vi "_Handle Error.vi"(4 "error in (no error)":errorcluster, 6 "Display Warning (T)":bool=TRUE, 7 "Display Error (T)":bool=TRUE) -> (3 "error?":bool)   [LabVIEW 2015]
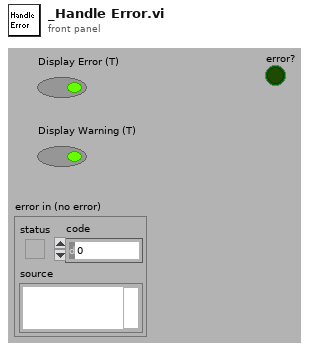
[diagram p1: front panel]
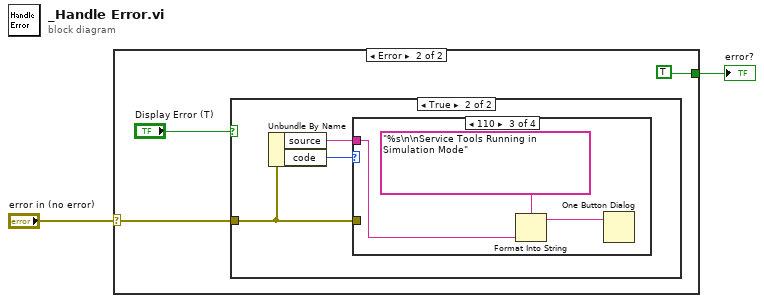
[diagram p0: block diagram]
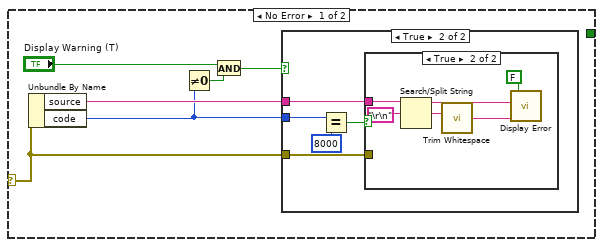
[diagram p2: hidden frame]
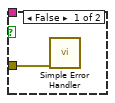
[diagram p4: hidden frame]
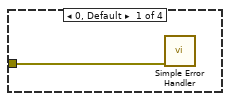
[diagram p6: hidden frame]
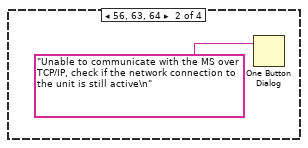
[diagram p7: hidden frame]
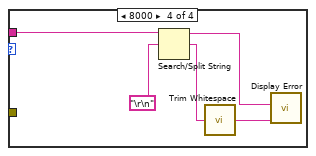
[diagram p8: hidden frame]
diagram:
  n1 = case shown="Error" "error in (no error)" {
    selector: "error in (no error)" -> [w3 w22]
    tunnel: [_ TRUE] -> w1
    frame No Error {
      n2 = Unbundle By Name(w3) -> ("source"=w5:string, "code"=w4:i32)
      n3 = Not Equal To 0?(x=w4) -> (x != 0?=w6:bool)
      n4 = And(x="Display Warning (T)", y=w6) -> (x .and. y?=w8:bool)
      n5 = case shown="True" w8 {
        tunnel: w3 -> [_ w11]
        tunnel: w5 -> [_ w10]
        tunnel: w4 -> [_ w9]
        frame False {
        }
        frame True {
          n6 = Equal?(x=w9, y=8000) -> (x = y?=w12:bool)
          n7 = case shown="True" w12 {
            tunnel: w11 -> [w14 _]
            tunnel: w10 -> [_ w20]
            frame False {
              n8 = call <vilib>:"Simple Error Handler.vi"("error in (no error)"=w14) -> ()  [unwired: 1 in, 8 out]
            }
            frame True {
              n9 = Search/Split String(string=w20, search string/char (-)="\r\n") -> (substring before match=w16:string, match + rest of string=w18:string)  [unwired: 2 out]
              n10 = call <vilib>:"Trim Whitespace.vi"("string"=w18) -> ("trimmed string"=w15:string)  [unwired: 1 in]
              n11 = call "Display Error.vi"("Cause :"=w15, "Source :"=w16, "Error? (T)"=FALSE) -> ()  [unwired: 1 in, 1 out]
            }
          }
        }
      }
    }
    frame Error {
      n12 = case shown="True" "Display Error (T)" {
        tunnel: w22 -> [_ w26]
        frame False {
        }
        frame True {
          n13 = Unbundle By Name(w26) -> ("source"=w25:string, "code"=w24:i32)
          n14 = case shown="110" w24 {
            tunnel: w26 -> [w27 _ _ _]
            tunnel: w25 -> [_ _ w30 w36]
            frame 0, Default {
              n15 = call <vilib>:"Simple Error Handler.vi"("error in (no error)"=w27) -> ()  [unwired: 1 in, 8 out]
            }
            frame 56, 63, 64 {
              n16 = One Button Dialog(message="Unable to communicate with the MS over TCP/IP, check if the network connection to the unit is still active\n") -> ()  [unwired: 1 in, 1 out]
            }
            frame 110 {
              n17 = Format Into String(format string="%s\n\nService Tools Running in Simulation Mode" ("message"), w30) -> (resulting string=w29:string)  [unwired: 2 in, 1 out]
              n18 = One Button Dialog(message=w29) -> ()  [unwired: 1 in, 1 out]
            }
            frame 8000 {
              n19 = Search/Split String(string=w36, search string/char (-)="\r\n") -> (substring before match=w33:string, match + rest of string=w34:string)  [unwired: 2 out]
              n20 = call <vilib>:"Trim Whitespace.vi"("string"=w34) -> ("trimmed string"=w32:string)  [unwired: 1 in]
              n21 = call "Display Error.vi"("Cause :"=w32, "Source :"=w33) -> ()  [unwired: 2 in, 1 out]
            }
          }
        }
      }
    }
  }
  "error?" <- w1
